vi "Keyboard_Main.vi"() -> ()   [LabVIEW 2023]
uses:
  <vilib>/event_ctls.llb/eventvkey.ctl
panel:
  in  "stop":bool
  in  "Tab Control":enum32{"User panel", "Status panel"}(tab)
  in  "Cluster commandes":T1={"Dia lamp"=TRUE, "Dia lamp intensity"=1689.1304347826087, "Objective"=2, "Light path"=2, "Z pos (µm)"=335593} {"Z pos (µm)" min=0 max=990000 step=100 scale=0.0..990000.0; "Light path" items=["1- Eyepiece"=1, "2- Right"=2, "3- Left + Eyepiece"=3, "4- Left"=4]; "Objective" items=["1- Target"=1, "2- PLAN APO 100X 1,45 Oil"=2, "3- Empty"=3, "4- Empty"=4, "5- Empty"=5, "6- Empty"=6]; "Dia lamp intensity" scale=0.0..2100.0}
  out "Cluster µscope":T2
  out "Z Position":dbl[](array[numeric]) format="%.6f"
  out "XY Positions":dbl[](array[numeric]) format="%.6f"
  in  "Keyboard":T4={"Array"=["Shift", "Shift+ Ctrl", "Shift", "Shift+ Ctrl", "Shift", "Shift+ Ctrl", "Shift", "Shift+ Ctrl", "Shift", "Shift+ Ctrl", "Shift", "Shift+ Ctrl", "Shift", "Shift+ Ctrl", "Shift", "Shift+ Ctrl"], "Array 2"=[enum."Up", enum."Up", enum."Down", enum."Down", enum."Left", enum."Left", enum."Right", enum."Right", enum."PageUp", enum."PageUp", enum."PageDown", enum."PageDown"], "Array 3"=[8.0, 8.0, 4.0, 4.0], "Array 4"=["X+", "X++", "X-", "X--", "Y+", "Y++", "Y-", "Y--", "Z+", "Z++", "Z-", "Z--", "Zobj+", "Zobj++", "Zobj-", "Zobj--"]}
  out "Nikon cluster":T5
  out "C-867-cluster":T6
  out "E-709-cluster":T7
  in  "error in (no error)":errorcluster
  out "error out":errorcluster
  in  "Relative XY\nmove (mm)":dbl
  in  "Relative Z obj\n move (au)":dbl
  in  "Relative Z\nmove (um)":dbl
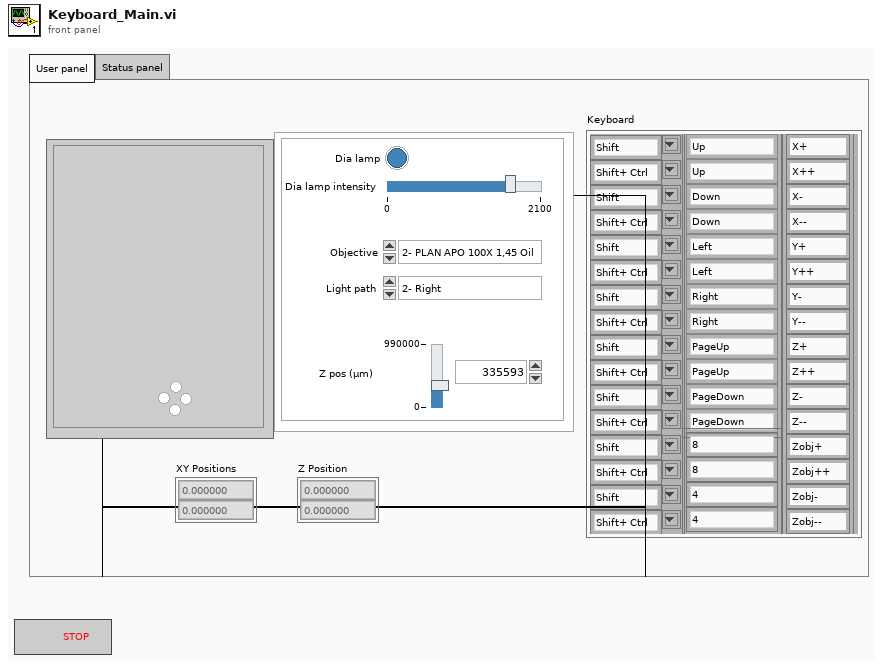
[diagram p1: front panel]
types:
  T1 = cluster{"Dia lamp":bool, "Dia lamp intensity":dbl, "Objective":i32, "Light path":u32, "Z pos (µm)":i32}
  T2 = cluster{"Eyepiece":bool, "Right":bool, "Left + Eyepiece":bool, "Left":bool}
  T3 = typedef "eventvkey.ctl" = enum16{"ASCII", "Enter", "Return", "Shift", "Ctrl", "Alt", "Cmd", "Opt", "Caps", "NumLock", "Clear", "Break", "Up", "Down", "Left", "Right", "Insert", "Delete", "Home", "End", "PageUp", "PageDown", "Escape", "Help", "Pause", "ScrollLock", "F1", "F2", "F3", "F4", "F5", "F6", "F7", "F8", "F9", "F10", "F11", "F12", "F13", "F14", "F15", "F16", "F17", "F18", "F19", "F20", "F21", "F22", "F23", "F24", "Play", "VolumeUp", "VolumeDown", "Mute", "Two Byte Char"}
  T4 = cluster{"Array":string[], "Array 2":T3[], "Array 3":dbl[], "Array 4":string[]}
  T5 = cluster{"reference out":refnum<k7>, "Nikon status cluster":cluster{"iNOSEPIECE":i32, "iLIGHTPATH":i32, "iDIA_LAMP_Switch":i32, "iDIA_LAMP_Pos":i32, "iZPOSITION":i32, "iPFS_SWITCH":i32, "iPFS_STATUS":i32, "iPFS_OFFSET":i32}}
  T6 = cluster{"Conn. \nAxis":string[], "Position":dbl[], "+/- movement\nrange":dbl[], "Servo status?":bool[]}
  T7 = cluster{"Conn. \nAxis":string[], "Positions":dbl[], "+/- movement\nrange":dbl[], "Servo status?":bool[]}
  T8 = cluster{"Shift":bool, "Ctrl":bool, "Alt":bool, "Cmd":bool, "Opt":bool}
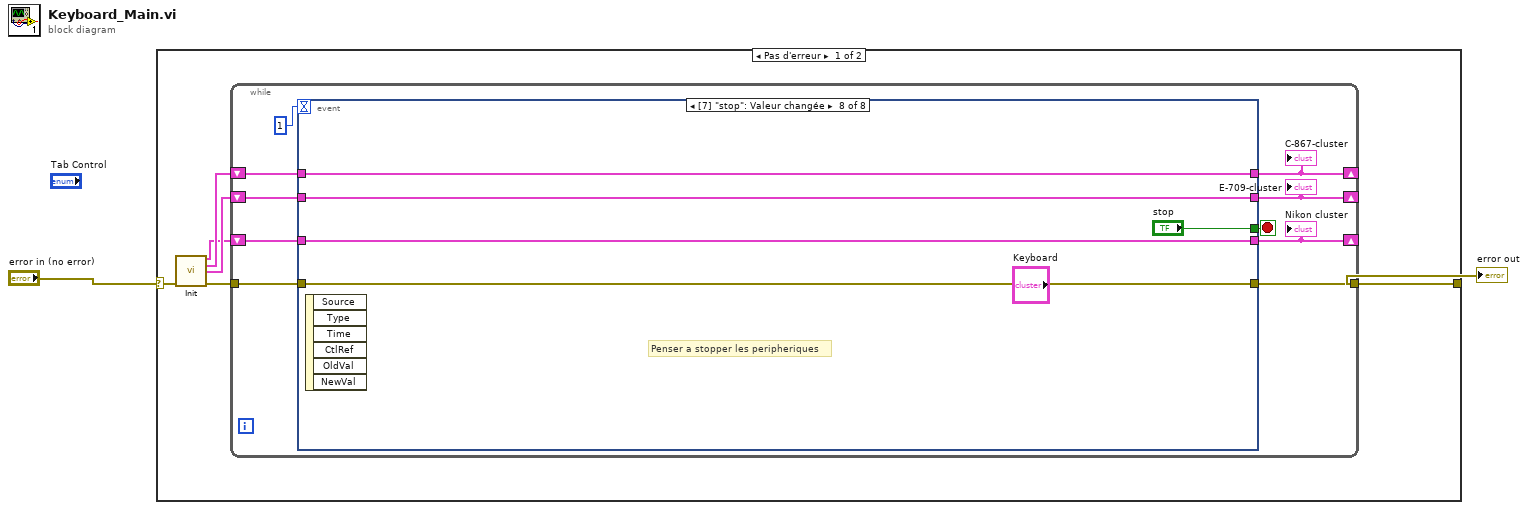
[diagram p0: block diagram]
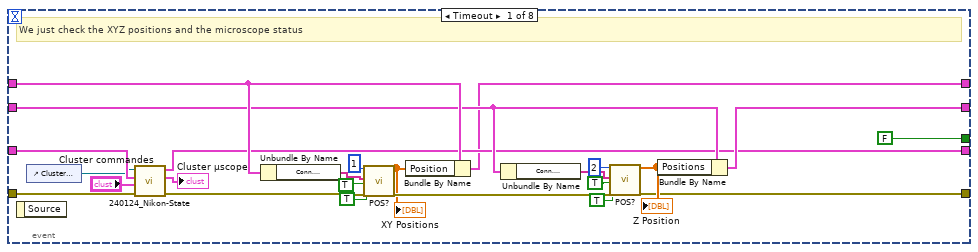
[diagram p2: hidden frame]
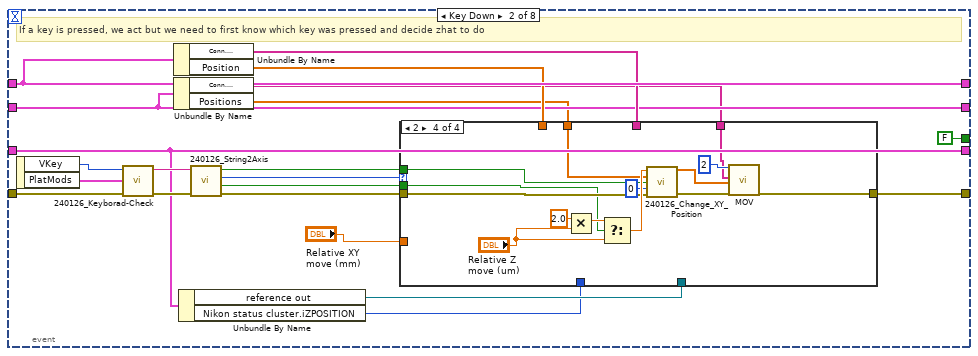
[diagram p3: hidden frame]
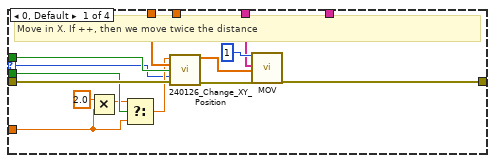
[diagram p4: hidden frame]
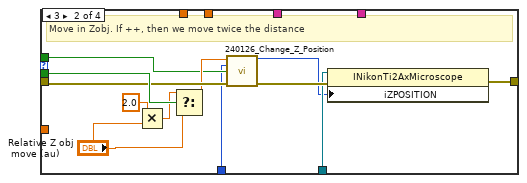
[diagram p5: hidden frame]
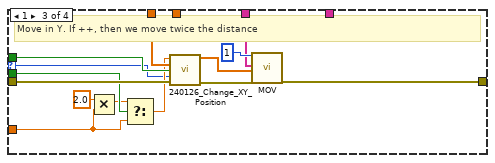
[diagram p6: hidden frame]
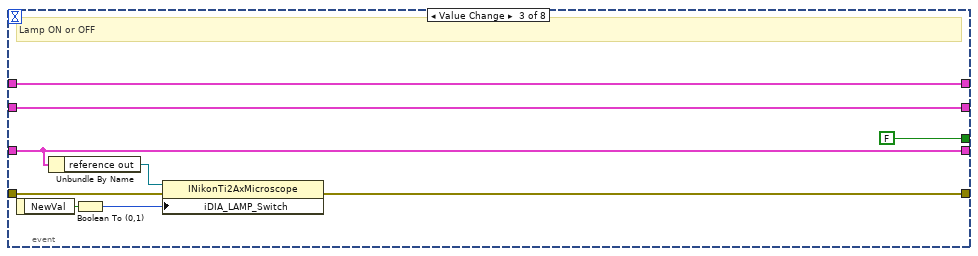
[diagram p7: hidden frame]
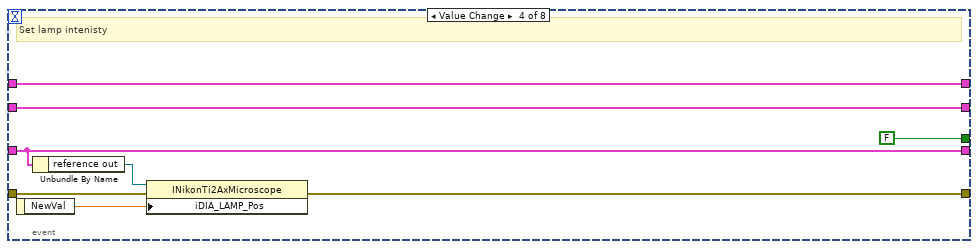
[diagram p8: hidden frame]
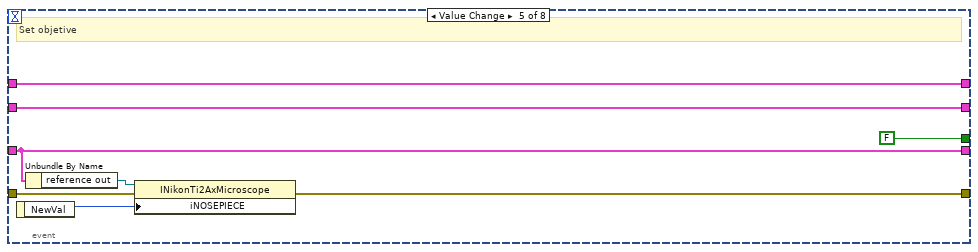
[diagram p9: hidden frame]
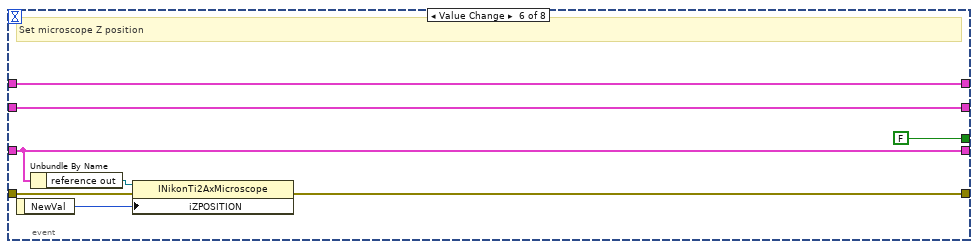
[diagram p10: hidden frame]
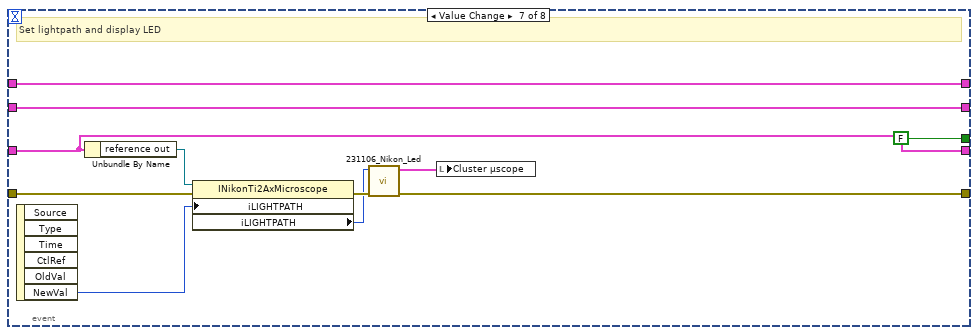
[diagram p11: hidden frame]
diagram:
  n1 = case shown="Pas d'erreur" "error in (no error)" {
    selector: "error in (no error)" -> [w8 w167]
    tunnel: [w3 w167] -> w1
    frame No Error {
      n2 = call "Init.vi"("error in (no error)"=w8) -> ("Nikon cluster"=w4:T5, "C-867-cluster"=w6:T6, "E-709-cluster"=w5:T7, "error out"=w7:errorcluster)  [unwired: 11 in]
      n3 = while {
        tunnel: [w17] -> w3
        tunnel: w7 -> [w16]
        shift-right: [w13] -> _
        shift-left: w4 -> [w15]
        shift-right: [w12] -> _
        shift-left: w6 -> [w11]
        shift-right: [w10] -> _
        shift-left: w5 -> [w9]
        stop <- w14 stop-if-true
        n4 = event shown="[7] \"stop\": Valeur changée" {
          selector: _ -> [_ _ _ _ _ _ _ _]
          dyn-events: _ -> [_ _ _ _ _ _ _ _]
          timeout: 1 -> [_ _ _ _ _ _ _ _]
          tunnel: [w19 w56 w123 w131 w140 w147 w159 w165] -> w17
          tunnel: w16 -> [w42 w59 w124 w132 w141 w150 w156 w165]
          tunnel: w15 -> [w40 w50 w122 w130 w139 w146 w158 w164]
          tunnel: [FALSE ("stop") FALSE ("stop") FALSE ("stop") FALSE ("stop") FALSE ("stop") FALSE ("stop") FALSE ("stop") "stop"] -> w14
          tunnel: [w21 w50 w122 w130 w139 w146 w158 w164] -> w13
          tunnel: [w20 w62 w119 w128 w136 w144 w152 w163] -> w12
          tunnel: w11 -> [w25 w62 w119 w128 w136 w144 w152 w163]
          tunnel: [w23 w46 w118 w127 w135 w143 w151 w162] -> w10
          tunnel: w9 -> [w24 w46 w118 w127 w135 w143 w151 w162]
          event Timeout {
            # "We just check the XYZ positions and the microscope status"
            n5 = event-data() -> ()  [unwired: 1 in, 1 out]
            n6 = control-ref of="Cluster commandes"() -> (w38:refnum<vi>)
            n7 = call "240124_Nikon-State.vi"("error in (no error)"=w42, "Cluster commandes"="Cluster commandes", "Nikon cluster in"=w40, "Cluster in"=w38) -> ("error out"=w33:errorcluster, "Cluster µscope"=→"Cluster µscope":T2, "Nikon cluster out"=w21:T5)  [unwired: 5 in]
            n8 = Unbundle By Name(w25) -> ("Conn. \nAxis"=w30:string[])
            n9 = call "POS?.vi"("System no."=1, "Axes to query"=w30, "All axes?"=TRUE, "Axis identifier?"=TRUE, "error in"=w33) -> ("Position"=w28:dbl[], "error out"=w32:errorcluster)  [unwired: 13 in]
            "XY Positions" <- w28
            n10 = Bundle By Name(cluster=w25, "Position"=w28) -> (w20:T6)
            n11 = Unbundle By Name(w24) -> ("Conn. \nAxis"=w37:string[])
            n12 = call "POS?.vi"("System no."=2, "Axes to query"=w37, "All axes?"=TRUE, "Axis identifier?"=TRUE, "error in"=w32) -> ("Position"=w34:dbl[], "error out"=w19:errorcluster)  [unwired: 13 in]
            "Z Position" <- w34
            n13 = Bundle By Name(cluster=w24, "Positions"=w34) -> (w23:T7)
          }
          event Key Down {
            # "If a key is pressed, we act but we need to first know which key was pressed and decide zhat to do"
            n14 = event-data() -> ("VKey"=w60:T3, "PlatMods"=w61:T8)  [unwired: 1 in]
            n15 = call "240126_Keyborad-Check.vi"("error in (no error)"=w59, "PlatMods"=w61, "VKey"=w60) -> ("error out"=w57:errorcluster, "String"=w58:string)  [unwired: 7 in]
            n16 = Unbundle By Name(w62) -> ("Conn. \nAxis"=w53:string[], "Position"=w54:dbl[])
            n17 = Unbundle By Name(w46) -> ("Conn. \nAxis"=w45:string[], "Positions"=w44:dbl[])
            n18 = Unbundle By Name(w50) -> ("reference out"=w49:refnum<k7>, "Nikon status cluster.iZPOSITION"=w48:i32)
            n19 = call "240126_String2Axis.vi"("error in (no error)"=w57, "String"=w58) -> ("error out"=w55:errorcluster, "++ ou --"=w51:bool, "Index"=w47:i32, "+-"=w52:bool)  [unwired: 6 in]
            n20 = case shown="2" w47 {
              selector: w47 -> [w65 _ w91 _]
              tunnel: [w76 w82 w102 w111] -> w56
              tunnel: w55 -> [w74 w85 w100 w110]
              tunnel: w54 -> [w73 _ w99 _]
              tunnel: w53 -> [w72 _ w98 _]
              tunnel: w52 -> [w70 w83 w96 w107]
              tunnel: w51 -> [w69 w89 w95 w106]
              tunnel: w49 -> [_ w80 _ _]
              tunnel: w48 -> [_ w78 _ _]
              tunnel: w45 -> [_ _ _ w109]
              tunnel: w44 -> [_ _ _ w108]
              tunnel: "Relative XY\nmove (mm)" -> [w64 _ w90 _]
              frame 0, Default {
                # "Move in X. If ++, then we move twice the distance"
                n21 = Multiply(x=2.0, y=w64) -> (x*y=w66:dbl)
                n22 = Select(t=w66, s=w69, f=w64) -> (s? t:f=w68:dbl)
                n23 = call "240126_Change_XY_Position.vi"("Relative move (mm)"=w68, "Position in"=w73, "-+ (FT)"=w70, "XY (0-1)"=w65, "error in (no error)"=w74) -> ("Position out"=w71:dbl[], "error out"=w75:errorcluster)  [unwired: 9 in]
                n24 = call "MOV.vi"("System no."=1, "Axes to move"=w72, "Position values"=w71, "error in"=w75) -> ("error out"=w76:errorcluster)  [unwired: 15 in]
              }
              frame 3 {
                # "Move in Zobj. If ++, then we move twice the distance"
                n25 = Multiply(x=2.0, y="Relative Z obj\n move (au)") -> (x*y=w88:dbl)
                n26 = Select(t=w88, s=w89, f="Relative Z obj\n move (au)") -> (s? t:f=w84:dbl)
                n27 = call "240126_Change_Z_Position.vi"("Relative move (au)"=w84, "Z position"=w78, "-+ (FT)"=w83, "error in (no error)"=w85) -> ("Z position out"=w79:u32, "error out"=w81:errorcluster)  [unwired: 10 in]
                n28 = property class="INikonTi2AxMicroscope"(reference=w80, error in=w81, "iZPOSITION"=w79) -> (error out=w82:errorcluster)  [unwired: 1 out]
              }
              frame 1 {
                # "Move in Y. If ++, then we move twice the distance"
                n29 = Multiply(x=2.0, y=w90) -> (x*y=w92:dbl)
                n30 = Select(t=w92, s=w95, f=w90) -> (s? t:f=w94:dbl)
                n31 = call "240126_Change_XY_Position.vi"("Relative move (mm)"=w94, "Position in"=w99, "-+ (FT)"=w96, "XY (0-1)"=w91, "error in (no error)"=w100) -> ("Position out"=w97:dbl[], "error out"=w101:errorcluster)  [unwired: 9 in]
                n32 = call "MOV.vi"("System no."=1, "Axes to move"=w98, "Position values"=w97, "error in"=w101) -> ("error out"=w102:errorcluster)  [unwired: 15 in]
              }
              frame 2 {
                n33 = Multiply(x=2.0, y="Relative Z\nmove (um)") -> (x*y=w117:dbl)
                n34 = Select(t=w117, s=w106, f="Relative Z\nmove (um)") -> (s? t:f=w115:dbl)
                n35 = call "240126_Change_XY_Position.vi"("Relative move (mm)"=w115, "Position in"=w108, "-+ (FT)"=w107, "XY (0-1)"=u8 0, "error in (no error)"=w110) -> ("Position out"=w114:dbl[], "error out"=w113:errorcluster)  [unwired: 9 in]
                n36 = call "MOV.vi"("System no."=2, "Axes to move"=w109, "Position values"=w114, "error in"=w113) -> ("error out"=w111:errorcluster)  [unwired: 15 in]
              }
            }
          }
          event "Cluster commandes.Dia lamp": Value Change {
            # "Lamp ON or OFF"
            n37 = event-data() -> ("NewVal"=w125:bool)  [unwired: 1 in]
            n38 = Unbundle By Name(w122) -> ("reference out"=w121:refnum<k7>)
            n39 = Boolean To (0,1)(Boolean=w125) -> (0, 1=w126:i16)
            n40 = property class="INikonTi2AxMicroscope"(reference=w121, error in=w124, "iDIA_LAMP_Switch"=w126) -> (error out=w123:errorcluster)  [unwired: 1 out]
          }
          event "Cluster commandes.Dia lamp intensity": Value Change {
            # "Set lamp intenisty"
            n41 = event-data() -> ("NewVal"=w134:dbl)  [unwired: 1 in]
            n42 = Unbundle By Name(w130) -> ("reference out"=w133:refnum<k7>)
            n43 = property class="INikonTi2AxMicroscope"(reference=w133, error in=w132, "iDIA_LAMP_Pos"=w134) -> (error out=w131:errorcluster)  [unwired: 1 out]
          }
          event "Cluster commandes.Objective": Value Change {
            # "Set objetive"
            n44 = event-data() -> ("NewVal"=w137:i32)  [unwired: 1 in]
            n45 = Unbundle By Name(w139) -> ("reference out"=w142:refnum<k7>)
            n46 = property class="INikonTi2AxMicroscope"(reference=w142, error in=w141, "iNOSEPIECE"=w137) -> (error out=w140:errorcluster)  [unwired: 1 out]
          }
          event "Cluster commandes.Z pos (µm)": Value Change {
            # "Set microscope Z position"
            n47 = event-data() -> ("NewVal"=w148:i32)  [unwired: 1 in]
            n48 = Unbundle By Name(w146) -> ("reference out"=w149:refnum<k7>)
            n49 = property class="INikonTi2AxMicroscope"(reference=w149, error in=w150, "iZPOSITION"=w148) -> (error out=w147:errorcluster)  [unwired: 1 out]
          }
          event "Cluster commandes.Light path": Value Change {
            # "Set lightpath and display LED"
            n50 = event-data() -> ("NewVal"=w155:u32)  [unwired: 1 in, 5 out]
            n51 = Unbundle By Name(w158) -> ("reference out"=w157:refnum<k7>)
            n52 = property class="INikonTi2AxMicroscope"(reference=w157, error in=w156, "iLIGHTPATH"=w155) -> (error out=w161:errorcluster, "iLIGHTPATH"=w160:i32)  [unwired: 1 out]
            n53 = call "231106_Nikon_Led.vi"("error in"=w161, "Light path"=w160) -> ("error out"=w159:errorcluster, "Cluster µscope"=w154:T2)  [unwired: 8 in]
            n54 = local write "Cluster µscope"(w154) -> ()
          }
          event "stop": Value Change {
            # "Penser a stopper les peripheriques"
            n55 = event-data() -> ()  [unwired: 1 in, 6 out]
          }
        }
        "C-867-cluster" <- w12
        "E-709-cluster" <- w10
        "Nikon cluster" <- w13
      }
    }
    frame Error {
    }
  }
  "error out" <- w1
